vi "Run.vi"(8 "error in (no error)":errorcluster, 11 "Channel in":refnum<class "Channel.lvclass">) -> (0 "error out":errorcluster, 3 "Channel out":refnum<class "Channel.lvclass">)   [LabVIEW 2018, in "Channel.lvclass"]
doc: "Run the channel"
uses:
  Channel.lvclass
  Channel.lvclass/Channel.ctl
  Simulated_CCD_Camera/Simulated Camera.lvclass/Simulated Camera.ctl
  State Machine/State Machine.lvclass
  Simulated_CCD_Camera/Simulated Camera.lvclass
  RxTx/RxTx.lvclass
  Header content/Header content.lvclass
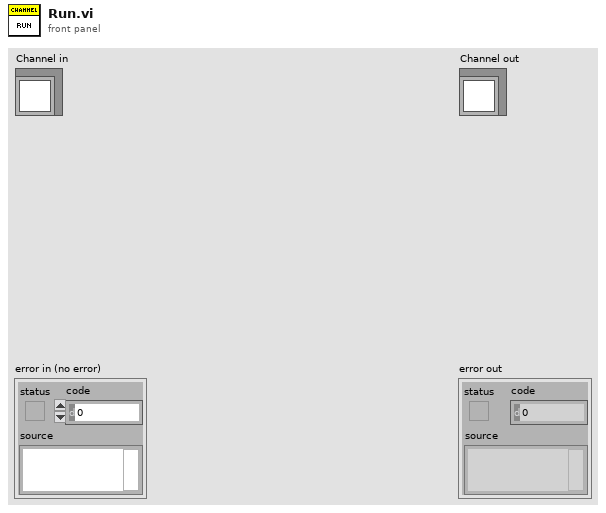
[diagram p1: front panel]
types:
  T1 = cluster{"PREAMP":u16, "READOUT_RATE":u16, "EM_GAIN":u16, "VERTICAL_SHIFT_SPEED":u16, "READ_MODE":u16, "FRAME_TRANSFER":bool, "VERTICAL_CLOCK_VOLTAGE":u16, "ACQUISITION_MODE":u16, "AD_CHANNEL":u16, "EM_MODE":u16, "SHUTTER_TTL":u16, "SHUTTER_OPENING_TIME":u16, "SHUTTER_CLOSING_TIME":u16, "SHUTTER_MODE":u16, "TRIGGER_MODE":u16, "VBIN":u16, "INITIAL_LINE":u16, "INITIAL_COLUMN":u16, "FINAL_LINE":u16, "FINAL_COLUMN":u16, "HBIN":u16}
  T2 = cluster{"CYCLES_DONE":u16, "LAST_IMAGE_NAME":string, "DISK_SPACE":u16, "FRAMES_DONE":u16, "CCD_STATUS":string, "CURRENT_TEMPERATURE":i16, "TEMPERATURE_STATUS":string, "FRAME_EXPOSURE_TIME":sgl, "ERROR":bool, "SERIAL_NUMBER":u16, "ACQUIRING":bool, "IMAGE_INDEX":u32, "SEQS_DONE":u16}
  T3 = cluster{"COOLER_POWER_STATUS":u16, "TEMP":i32, "EXPTIME":dbl, "#FRAMES":u32, "#CYCLES":u32, "#SEQS":u32, "WAVEPLATE_POS":u16}
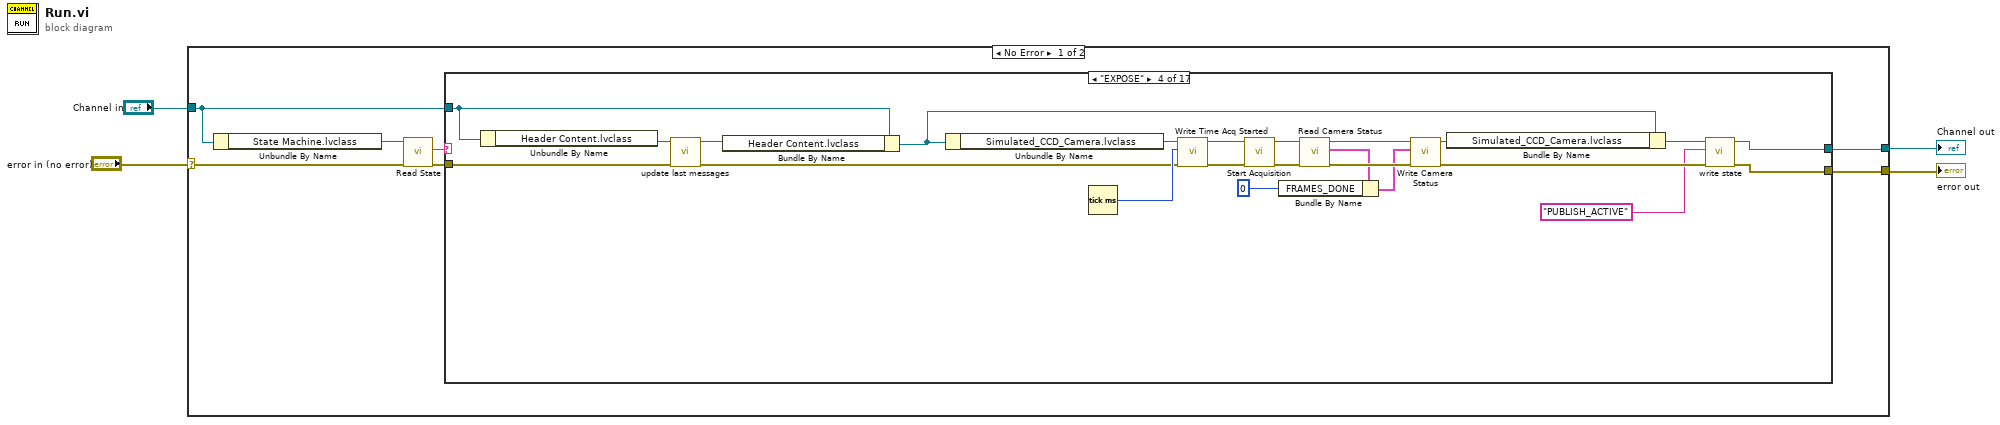
[diagram p0: block diagram]
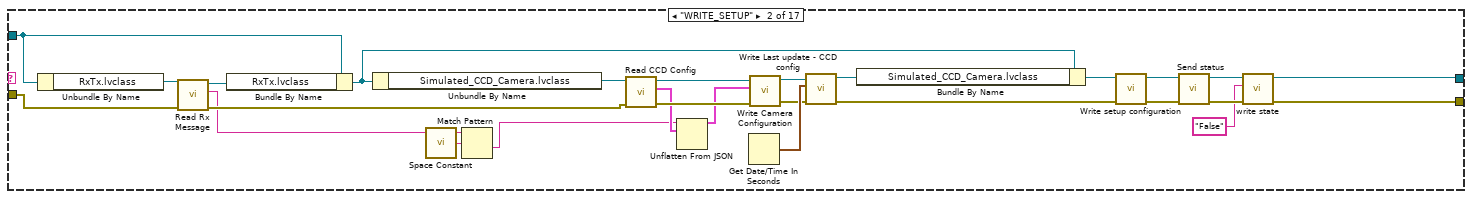
[diagram p3: hidden frame]
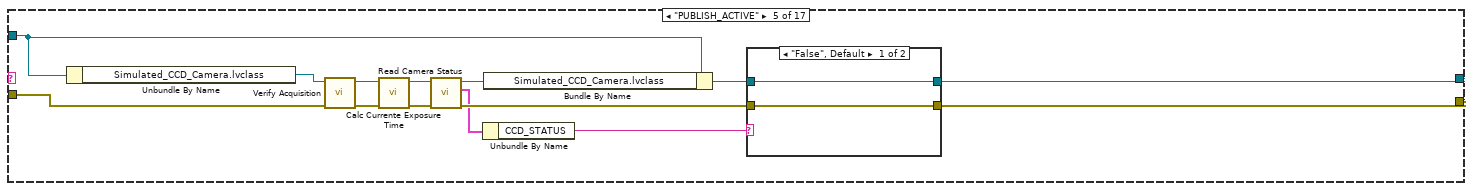
[diagram p5: hidden frame]
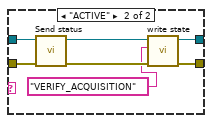
[diagram p6: hidden frame]
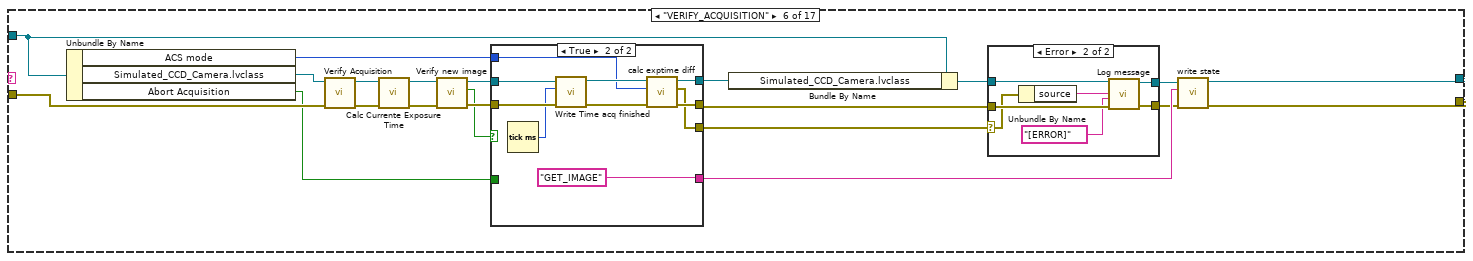
[diagram p7: hidden frame]
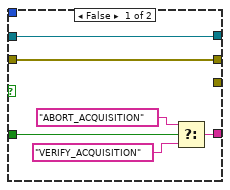
[diagram p9: hidden frame]
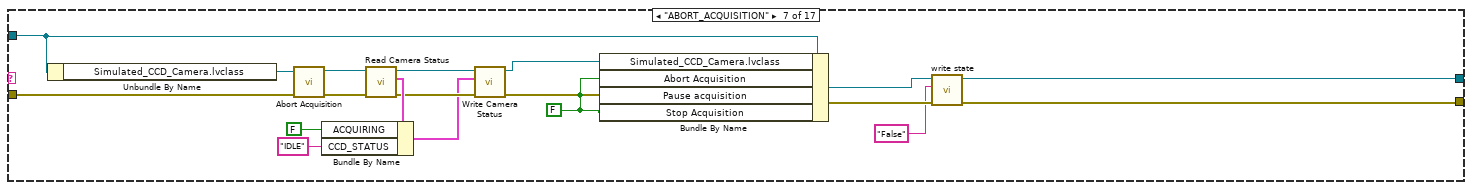
[diagram p10: hidden frame]
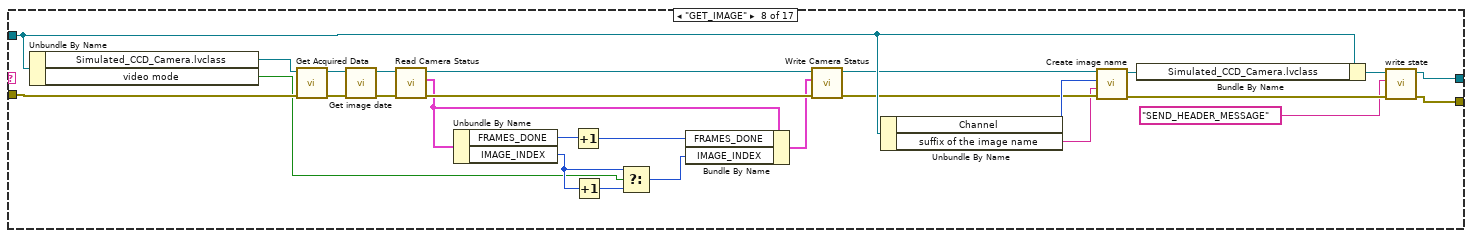
[diagram p11: hidden frame]
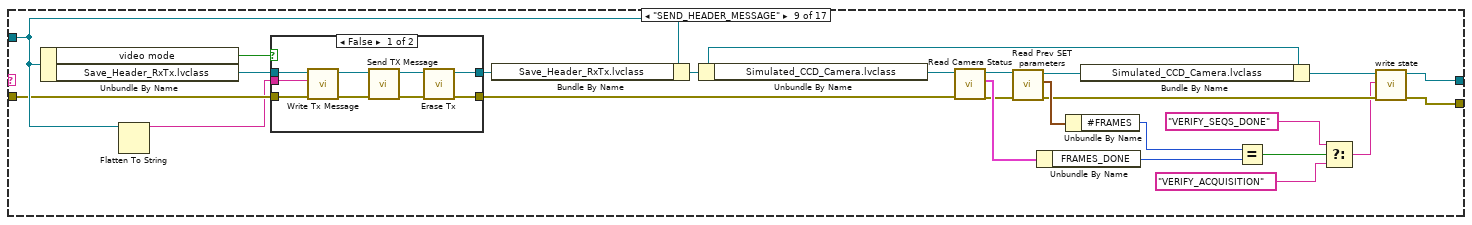
[diagram p12: hidden frame]
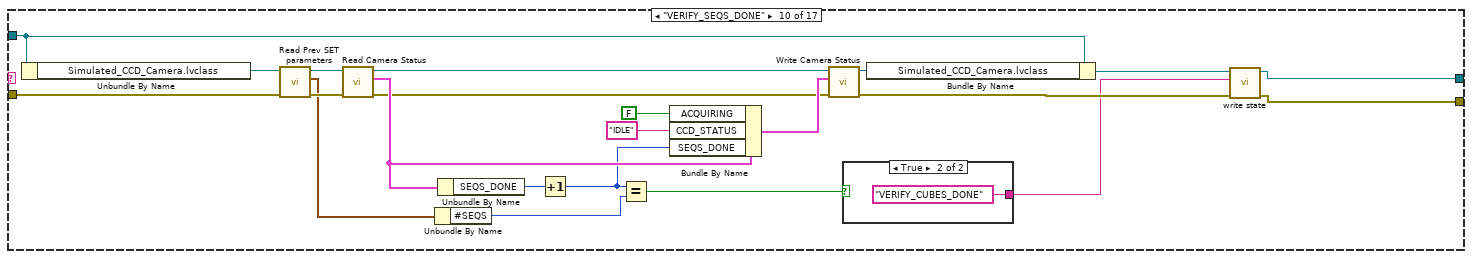
[diagram p14: hidden frame]
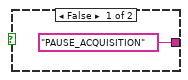
[diagram p15: hidden frame]
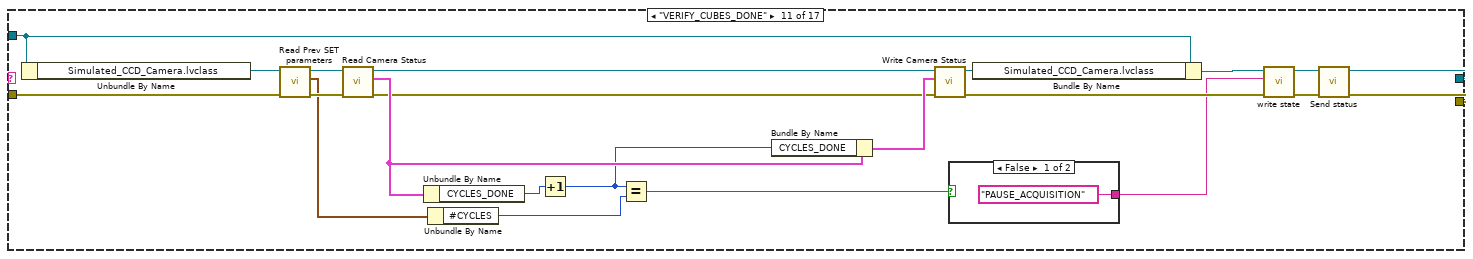
[diagram p16: hidden frame]
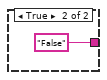
[diagram p17: hidden frame]
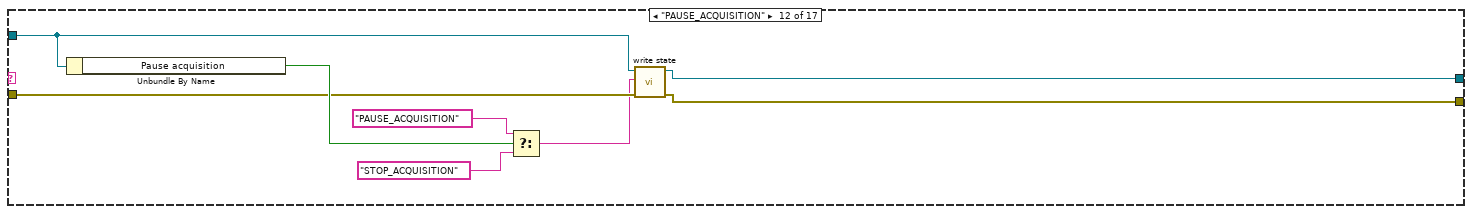
[diagram p18: hidden frame]
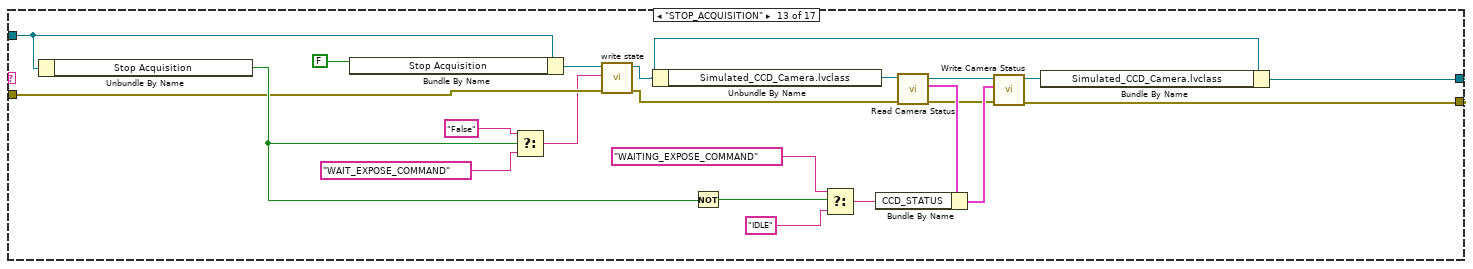
[diagram p19: hidden frame]
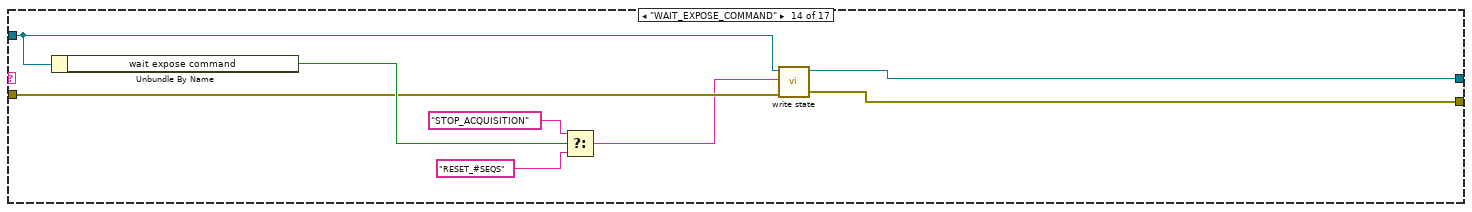
[diagram p20: hidden frame]
diagram:
  n1 = case shown="No Error" "error in (no error)" {
    selector: "error in (no error)" -> [w7 w427]
    tunnel: [w11 w427] -> w3
    tunnel: [w9 w426] -> w1
    tunnel: "Channel in" -> [w10 w426]
    frame No Error {
      n2 = Unbundle By Name(w10) -> ("State Machine.lvclass"=w8:refnum<class "State Machine.lvclass">)
      n3 = call-dynamic "Read State.vi"("error in (no error)"=w7, "State Machine in"=w8) -> ("error out"=w6:errorcluster, "State"=w5:string)  [unwired: 7 in, 1 out]
      n4 = case shown="\"EXPOSE\"" w5 {
        tunnel: w6 -> [w12 w38 w41 w56 w76 w105 w143 w179 w189 w227 w252 w266 w272 w296 w304 w322 w339]
        tunnel: [w12 w23 w41 w47 w72 w101 w136 w153 w180 w215 w244 w265 w279 w295 w301 w322 w329] -> w11
        tunnel: [w13 w24 w42 w48 w73 w102 w137 w154 w181 w216 w245 w264 w280 w294 w302 w323 w330] -> w9
        tunnel: w10 -> [w13 w40 w42 w55 w79 w109 w142 w172 w191 w231 w258 w267 w292 w297 w307 w323 w341]
        frame "False", Default {
        }
        frame "WRITE_SETUP" {
          n5 = Unbundle By Name(w40) -> ("RxTx.lvclass"=w39:refnum<class "RxTx.lvclass">)
          n6 = call "Read Rx Message.vi"("error in (no error)"=w38, "RxTx in"=w39) -> ("error out"=w33:errorcluster, "Rx Message"=w15:string, "RxTx out"=w37:refnum<class "RxTx.lvclass">)  [unwired: 7 in]
          n7 = Bundle By Name(cluster=w40, "RxTx.lvclass"=w37) -> (w28:refnum<class "Channel.lvclass">)
          n8 = Unbundle By Name(w28) -> ("Simulated_CCD_Camera.lvclass"=w36:refnum<class "Simulated Camera.lvclass">)
          n9 = call <vilib>:"Space Constant.vi"() -> ("String"=w16:string)
          n10 = Match Pattern(string=w15, regular expression=w16) -> (after substring=w14:string)  [unwired: 1 in, 3 out]
          n11 = call "Read CCD Config.vi"("error in (no error)"=w33, "CCDCamera in"=w36) -> ("error out"=w34:errorcluster, "CCD Config"=w32:T1, "CCDCamera out"=w35:refnum<class "Simulated Camera.lvclass">)  [unwired: 7 in]
          n12 = Unflatten From JSON(JSON string=w14, type and defaults=w32) -> (value=w31:T1)  [unwired: 5 in, 1 out]
          n13 = Get Date/Time In Seconds() -> (seconds since 1Jan1904=w30:timestamp)
          n14 = call-dynamic "Write Camera Configuration.vi"("error in (no error)"=w34, "CCD Config"=w31, "CCDCamera in"=w35) -> ("error out"=w21:errorcluster, "CCDCamera out"=w22:refnum<class "Simulated Camera.lvclass">)  [unwired: 7 in]
          n15 = call-dynamic "Write Last update - CCD config.vi"("error in (no error)"=w21, "Last update - CCD config"=w30, "Simulated_CCD_Camera in"=w22) -> ("error out"=w19:errorcluster, "Simulated_CCD_Camera out"=w29:refnum<class "Simulated Camera.lvclass">)  [unwired: 7 in]
          n16 = Bundle By Name(cluster=w28, "Simulated_CCD_Camera.lvclass"=w29) -> (w20:refnum<class "Channel.lvclass">)
          n17 = call "Write setup configuration.vi"("error in (no error)"=w19, "Channel in"=w20) -> ("error out"=w18:errorcluster, "Channel out"=w17:refnum<class "Channel.lvclass">)  [unwired: 8 in]
          n18 = call "Send status.vi"("error in (no error)"=w18, "Channel in"=w17) -> ("error out"=w26:errorcluster, "Channel out"=w27:refnum<class "Channel.lvclass">)  [unwired: 8 in]
          n19 = call "write state.vi"("error in (no error)"=w26, "state"="False", "Channel in"=w27) -> ("error out"=w23:errorcluster, "Channel out"=w24:refnum<class "Channel.lvclass">)  [unwired: 7 in]
        }
        frame "---------------------------------" {
        }
        frame "EXPOSE" {
          n20 = Unbundle By Name(w55) -> ("Header Content.lvclass"=w57:refnum<class "Header content.lvclass">)
          n21 = call "update last messages.vi"("error in (no error)"=w56, "Header content in"=w57) -> ("error out"=w53:errorcluster, "Header content out"=w54:refnum<class "Header content.lvclass">)  [unwired: 8 in]
          n22 = Bundle By Name(cluster=w55, "Header Content.lvclass"=w54) -> (w52:refnum<class "Channel.lvclass">)
          n23 = Unbundle By Name(w52) -> ("Simulated_CCD_Camera.lvclass"=w65:refnum<class "Simulated Camera.lvclass">)
          n24 = Tick Count (ms)() -> (millisecond timer value=w64:u32)
          n25 = call "Write Time Acq Started.vi"("error in (no error)"=w53, "Time Acq Started"=w64, "Simulated_CCD_Camera in"=w65) -> ("error out"=w43:errorcluster, "Simulated_CCD_Camera out"=w46:refnum<class "Simulated Camera.lvclass">)  [unwired: 7 in]
          n26 = call-dynamic "Start Acquisition.vi"("error in (no error)"=w43, "CCDCamera in"=w46) -> ("error out"=w44:errorcluster, "CCDCamera out"=w45:refnum<class "Simulated Camera.lvclass">)  [unwired: 8 in]
          n27 = call "Read Camera Status.vi"("error in (no error)"=w44, "CCDCamera in"=w45) -> ("error out"=w62:errorcluster, "Camera Status"=w60:T2, "CCDCamera out"=w61:refnum<class "Simulated Camera.lvclass">)  [unwired: 7 in]
          n28 = Bundle By Name(cluster=w60, "FRAMES_DONE"=u16 0) -> (w59:T2)
          n29 = call "Write Camera Status.vi"("error in (no error)"=w62, "Camera Status"=w59, "CCDCamera in"=w61) -> ("error out"=w50:errorcluster, "CCDCamera out"=w63:refnum<class "Simulated Camera.lvclass">)  [unwired: 7 in]
          n30 = Bundle By Name(cluster=w52, "Simulated_CCD_Camera.lvclass"=w63) -> (w51:refnum<class "Channel.lvclass">)
          n31 = call "write state.vi"("error in (no error)"=w50, "state"="PUBLISH_ACTIVE", "Channel in"=w51) -> ("error out"=w47:errorcluster, "Channel out"=w48:refnum<class "Channel.lvclass">)  [unwired: 7 in]
        }
        frame "PUBLISH_ACTIVE" {
          n32 = Unbundle By Name(w79) -> ("Simulated_CCD_Camera.lvclass"=w77:refnum<class "Simulated Camera.lvclass">)
          n33 = call-dynamic "Verify Acquisition.vi"("error in (no error)"=w76, "CCDCamera in"=w77) -> ("error out"=w78:errorcluster, "CCDCamera out"=w75:refnum<class "Simulated Camera.lvclass">)  [unwired: 8 in]
          n34 = call-dynamic "Calc Currente Exposure Time.vi"("error in (no error)"=w78, "CCDCamera in"=w75) -> ("error out"=w71:errorcluster, "CCDCamera out"=w70:refnum<class "Simulated Camera.lvclass">)  [unwired: 8 in]
          n35 = call "Read Camera Status.vi"("error in (no error)"=w71, "CCDCamera in"=w70) -> ("error out"=w68:errorcluster, "Camera Status"=w67:T2, "CCDCamera out"=w69:refnum<class "Simulated Camera.lvclass">)  [unwired: 7 in]
          n36 = Unbundle By Name(w67) -> ("CCD_STATUS"=w66:string)
          n37 = Bundle By Name(cluster=w79, "Simulated_CCD_Camera.lvclass"=w69) -> (w74:refnum<class "Channel.lvclass">)
          n38 = case shown="\"False\", Default" w66 {
            tunnel: w74 -> [w81 w84]
            tunnel: [w81 w88] -> w73
            tunnel: [w80 w87] -> w72
            tunnel: w68 -> [w80 w83]
            frame "False", Default {
            }
            frame "ACTIVE" {
              n39 = call "Send status.vi"("error in (no error)"=w83, "Channel in"=w84) -> ("error out"=w86:errorcluster, "Channel out"=w85:refnum<class "Channel.lvclass">)  [unwired: 8 in]
              n40 = call "write state.vi"("error in (no error)"=w86, "state"="VERIFY_ACQUISITION", "Channel in"=w85) -> ("error out"=w87:errorcluster, "Channel out"=w88:refnum<class "Channel.lvclass">)  [unwired: 7 in]
            }
          }
        }
        frame "VERIFY_ACQUISITION" {
          n41 = Unbundle By Name(w109) -> ("ACS mode"=w94:u16, "Simulated_CCD_Camera.lvclass"=w106:refnum<class "Simulated Camera.lvclass">, "Abort Acquisition"=w97:bool)
          n42 = call-dynamic "Verify Acquisition.vi"("error in (no error)"=w105, "CCDCamera in"=w106) -> ("error out"=w107:errorcluster, "CCDCamera out"=w104:refnum<class "Simulated Camera.lvclass">)  [unwired: 8 in]
          n43 = call-dynamic "Calc Currente Exposure Time.vi"("error in (no error)"=w107, "CCDCamera in"=w104) -> ("error out"=w108:errorcluster, "CCDCamera out"=w103:refnum<class "Simulated Camera.lvclass">)  [unwired: 8 in]
          n44 = call-dynamic "Verify new image.vi"("error in (no error)"=w108, "CCDCamera in"=w103) -> ("error out"=w99:errorcluster, "New Images ?"=w96:bool, "CCDCamera out"=w100:refnum<class "Simulated Camera.lvclass">)  [unwired: 7 in]
          n45 = case shown="True" w96 {
            tunnel: w100 -> [w124 w134]
            tunnel: w99 -> [w123 w133]
            tunnel: [w124 w128] -> w98
            tunnel: [w123 w129] -> w90
            tunnel: w97 -> [w120 _]
            tunnel: [w119 "GET_IMAGE"] -> w95
            tunnel: w94 -> [_ w126]
            tunnel: [_ w125] -> w89
            frame False {
              n46 = Select(t="ABORT_ACQUISITION", s=w120, f="VERIFY_ACQUISITION") -> (s? t:f=w119:string)
            }
            frame True {
              n47 = Tick Count (ms)() -> (millisecond timer value=w131:u32)
              n48 = call "Write Time acq finished.vi"("error in (no error)"=w133, "Time acq finished"=w131, "Simulated_CCD_Camera in"=w134) -> ("error out"=w130:errorcluster, "Simulated_CCD_Camera out"=w127:refnum<class "Simulated Camera.lvclass">)  [unwired: 7 in]
              n49 = call "calc exptime diff.vi"("error in (no error)"=w130, "ACS mode"=w126, "Simulated_CCD_Camera in"=w127) -> (0:"error out"=w129:errorcluster, 2:"error out"=w125:errorcluster, "Simulated_CCD_Camera out"=w128:refnum<class "Simulated Camera.lvclass">)  [unwired: 6 in]
            }
          }
          n50 = Bundle By Name(cluster=w109, "Simulated_CCD_Camera.lvclass"=w98) -> (w93:refnum<class "Channel.lvclass">)
          n51 = case shown="Error" w89 {
            selector: w89 -> [_ w113]
            tunnel: w93 -> [w111 w118]
            tunnel: [w111 w117] -> w92
            tunnel: [w110 w116] -> w91
            tunnel: w90 -> [w110 w115]
            frame No Error {
            }
            frame Error {
              n52 = Unbundle By Name(w113) -> ("source"=w112:string)
              n53 = call "Log message.vi"("error in (no error)"=w115, "message type"="[ERROR]", "String"=w112, "Channel in"=w118) -> ("error out"=w116:errorcluster, "Channel out"=w117:refnum<class "Channel.lvclass">)  [unwired: 6 in]
            }
          }
          n54 = call "write state.vi"("error in (no error)"=w91, "state"=w95, "Channel in"=w92) -> ("error out"=w101:errorcluster, "Channel out"=w102:refnum<class "Channel.lvclass">)  [unwired: 7 in]
        }
        frame "ABORT_ACQUISITION" {
          w135 = FALSE ("Acquiring")
          n55 = Unbundle By Name(w142) -> ("Simulated_CCD_Camera.lvclass"=w144:refnum<class "Simulated Camera.lvclass">)
          n56 = call-dynamic "Abort Acquisition.vi"("error in (no error)"=w143, "CCDCamera in"=w144) -> ("error out"=w149:errorcluster, "CCDCamera out"=w150:refnum<class "Simulated Camera.lvclass">)  [unwired: 8 in]
          n57 = call "Read Camera Status.vi"("error in (no error)"=w149, "CCDCamera in"=w150) -> ("error out"=w147:errorcluster, "Camera Status"=w152:T2, "CCDCamera out"=w148:refnum<class "Simulated Camera.lvclass">)  [unwired: 7 in]
          n58 = Bundle By Name(cluster=w152, "ACQUIRING"=FALSE ("Acquiring"), "CCD_STATUS"="IDLE" ("STATUS")) -> (w146:T2)
          n59 = call "Write Camera Status.vi"("error in (no error)"=w147, "Camera Status"=w146, "CCDCamera in"=w148) -> ("error out"=w139:errorcluster, "CCDCamera out"=w141:refnum<class "Simulated Camera.lvclass">)  [unwired: 7 in]
          n60 = Bundle By Name(cluster=w142, "Simulated_CCD_Camera.lvclass"=w141, "Abort Acquisition"=w135, "Pause acquisition"=w135, "Stop Acquisition"=w135) -> (w140:refnum<class "Channel.lvclass">)
          n61 = call "write state.vi"("error in (no error)"=w139, "state"="False", "Channel in"=w140) -> ("error out"=w136:errorcluster, "Channel out"=w137:refnum<class "Channel.lvclass">)  [unwired: 7 in]
        }
        frame "GET_IMAGE" {
          n62 = Unbundle By Name(w172) -> ("Simulated_CCD_Camera.lvclass"=w161:refnum<class "Simulated Camera.lvclass">, "video mode"=w158:bool)
          n63 = call-dynamic "Get Acquired Data.vi"("error in (no error)"=w179, "CCDCamera in"=w161) -> ("error out"=w164:errorcluster, "CCDCamera out"=w167:refnum<class "Simulated Camera.lvclass">)  [unwired: 8 in]
          n64 = call-dynamic "Get image date.vi"("error in (no error)"=w164, "Simulated_CCD_Camera in"=w167) -> ("error out"=w165:errorcluster, "Simulated_CCD_Camera out"=w166:refnum<class "Simulated Camera.lvclass">)  [unwired: 8 in]
          n65 = call "Read Camera Status.vi"("error in (no error)"=w165, "CCDCamera in"=w166) -> ("error out"=w178:errorcluster, "Camera Status"=w174:T2, "CCDCamera out"=w177:refnum<class "Simulated Camera.lvclass">)  [unwired: 7 in]
          n66 = Unbundle By Name(w174) -> ("FRAMES_DONE"=w176:u16, "IMAGE_INDEX"=w159:u32)
          n67 = Increment(x=w176) -> (x+1=w162:u16)
          n68 = Increment(x=w159) -> (x+1=w160:u32)
          n69 = Select(t=w159, s=w158, f=w160) -> (s? t:f=w163:u32)
          n70 = Bundle By Name(cluster=w174, "FRAMES_DONE"=w162, "IMAGE_INDEX"=w163) -> (w175:T2)
          n71 = call "Write Camera Status.vi"("error in (no error)"=w178, "Camera Status"=w175, "CCDCamera in"=w177) -> ("error out"=w169:errorcluster, "CCDCamera out"=w170:refnum<class "Simulated Camera.lvclass">)  [unwired: 7 in]
          n72 = Unbundle By Name(w172) -> ("Channel"=w171:u8, "suffix of the image name"=w168:string)
          n73 = call "Create image name.vi"("error in (no error)"=w169, "Suffix"=w168, "Channel"=w171, "Simulated_CCD_Camera in"=w170) -> ("error out"=w156:errorcluster, "Simulated_CCD_Camera out"=w173:refnum<class "Simulated Camera.lvclass">)  [unwired: 6 in]
          n74 = Bundle By Name(cluster=w172, "Simulated_CCD_Camera.lvclass"=w173) -> (w157:refnum<class "Channel.lvclass">)
          n75 = call "write state.vi"("error in (no error)"=w156, "state"="SEND_HEADER_MESSAGE", "Channel in"=w157) -> ("error out"=w153:errorcluster, "Channel out"=w154:refnum<class "Channel.lvclass">)  [unwired: 7 in]
        }
        frame "SEND_HEADER_MESSAGE" {
          n76 = Unbundle By Name(w191) -> ("video mode"=w185:bool, "Save_Header_RxTx.lvclass"=w190:refnum<class "RxTx.lvclass">)
          n77 = Flatten To String(anything=w191) -> (data string=w186:string)  [unwired: 3 in, 2 out]
          n78 = case shown="False" w185 {
            tunnel: w190 -> [w212 w214]
            tunnel: w189 -> [w209 w213]
            tunnel: [w207 w214] -> w188
            tunnel: [w205 w213] -> w187
            tunnel: w186 -> [w204 _]
            frame False {
              n79 = call "Write Tx Message.vi"("error in (no error)"=w209, "Tx Message"=w204, "RxTx in"=w212) -> ("error out"=w210:errorcluster, "RxTx out"=w211:refnum<class "RxTx.lvclass">)  [unwired: 7 in]
              n80 = call "Send TX Message.vi"("error in (no error)"=w210, "RxTx in"=w211) -> ("error out"=w206:errorcluster, "RxTx out"=w208:refnum<class "RxTx.lvclass">)  [unwired: 8 in]
              n81 = call "Erase Tx.vi"("error in (no error)"=w206, "RxTx in"=w208) -> ("error out"=w205:errorcluster, "RxTx out"=w207:refnum<class "RxTx.lvclass">)  [unwired: 8 in]
            }
            frame True {
            }
          }
          n82 = Bundle By Name(cluster=w191, "Save_Header_RxTx.lvclass"=w188) -> (w201:refnum<class "Channel.lvclass">)
          n83 = Unbundle By Name(w201) -> ("Simulated_CCD_Camera.lvclass"=w198:refnum<class "Simulated Camera.lvclass">)
          n84 = call "Read Camera Status.vi"("error in (no error)"=w187, "CCDCamera in"=w198) -> ("error out"=w194:errorcluster, "Camera Status"=w197:T2, "CCDCamera out"=w196:refnum<class "Simulated Camera.lvclass">)  [unwired: 7 in]
          n85 = call-dynamic "Read Prev SET parameters.vi"("error in (no error)"=w194, "Simulated_CCD_Camera in"=w196) -> ("error out"=w183:errorcluster, "Prev SET parameters"=w193:T3, "Simulated_CCD_Camera out"=w195:refnum<class "Simulated Camera.lvclass">)  [unwired: 7 in]
          n86 = Unbundle By Name(w197) -> ("FRAMES_DONE"=w203:u16)
          n87 = Unbundle By Name(w193) -> ("#FRAMES"=w192:u32)
          n88 = Bundle By Name(cluster=w201, "Simulated_CCD_Camera.lvclass"=w195) -> (w184:refnum<class "Channel.lvclass">)
          n89 = Equal?(x=w192, y=w203) -> (x = y?=w202:bool)
          n90 = Select(t="VERIFY_SEQS_DONE", s=w202, f="VERIFY_ACQUISITION") -> (s? t:f=w182:string)
          n91 = call "write state.vi"("error in (no error)"=w183, "state"=w182, "Channel in"=w184) -> ("error out"=w180:errorcluster, "Channel out"=w181:refnum<class "Channel.lvclass">)  [unwired: 7 in]
        }
        frame "VERIFY_SEQS_DONE" {
          n92 = Unbundle By Name(w231) -> ("Simulated_CCD_Camera.lvclass"=w230:refnum<class "Simulated Camera.lvclass">)
          n93 = call-dynamic "Read Prev SET parameters.vi"("error in (no error)"=w227, "Simulated_CCD_Camera in"=w230) -> ("error out"=w228:errorcluster, "Prev SET parameters"=w226:T3, "Simulated_CCD_Camera out"=w229:refnum<class "Simulated Camera.lvclass">)  [unwired: 7 in]
          n94 = call "Read Camera Status.vi"("error in (no error)"=w228, "CCDCamera in"=w229) -> ("error out"=w222:errorcluster, "Camera Status"=w236:T2, "CCDCamera out"=w223:refnum<class "Simulated Camera.lvclass">)  [unwired: 7 in]
          n95 = Unbundle By Name(w226) -> ("#SEQS"=w225:u32)
          n96 = Unbundle By Name(w236) -> ("SEQS_DONE"=w235:u16)
          n97 = Increment(x=w235) -> (x+1=w233:u16)
          n98 = Equal?(x=w233, y=w225) -> (x = y?=w232:bool)
          n99 = Bundle By Name(cluster=w236, "ACQUIRING"=FALSE, "CCD_STATUS"="IDLE", "SEQS_DONE"=w233) -> (w234:T2)
          n100 = call "Write Camera Status.vi"("error in (no error)"=w222, "Camera Status"=w234, "CCDCamera in"=w223) -> ("error out"=w218:errorcluster, "CCDCamera out"=w224:refnum<class "Simulated Camera.lvclass">)  [unwired: 7 in]
          n101 = case shown="True" w232 {
            tunnel: ["PAUSE_ACQUISITION" "VERIFY_CUBES_DONE"] -> w217
            frame False {
            }
            frame True {
            }
          }
          n102 = Bundle By Name(cluster=w231, "Simulated_CCD_Camera.lvclass"=w224) -> (w219:refnum<class "Channel.lvclass">)
          n103 = call "write state.vi"("error in (no error)"=w218, "state"=w217, "Channel in"=w219) -> ("error out"=w215:errorcluster, "Channel out"=w216:refnum<class "Channel.lvclass">)  [unwired: 7 in]
        }
        frame "VERIFY_CUBES_DONE" {
          n104 = Unbundle By Name(w258) -> ("Simulated_CCD_Camera.lvclass"=w255:refnum<class "Simulated Camera.lvclass">)
          n105 = call-dynamic "Read Prev SET parameters.vi"("error in (no error)"=w252, "Simulated_CCD_Camera in"=w255) -> ("error out"=w253:errorcluster, "Prev SET parameters"=w251:T3, "Simulated_CCD_Camera out"=w254:refnum<class "Simulated Camera.lvclass">)  [unwired: 7 in]
          n106 = call "Read Camera Status.vi"("error in (no error)"=w253, "CCDCamera in"=w254) -> ("error out"=w256:errorcluster, "Camera Status"=w260:T2, "CCDCamera out"=w257:refnum<class "Simulated Camera.lvclass">)  [unwired: 7 in]
          n107 = Unbundle By Name(w260) -> ("CYCLES_DONE"=w246:u16)
          n108 = Unbundle By Name(w251) -> ("#CYCLES"=w250:u32)
          n109 = Increment(x=w246) -> (x+1=w248:u16)
          n110 = Equal?(x=w248, y=w250) -> (x = y?=w247:bool)
          n111 = Bundle By Name(cluster=w260, "CYCLES_DONE"=w248) -> (w259:T2)
          n112 = call "Write Camera Status.vi"("error in (no error)"=w256, "Camera Status"=w259, "CCDCamera in"=w257) -> ("error out"=w240:errorcluster, "CCDCamera out"=w249:refnum<class "Simulated Camera.lvclass">)  [unwired: 7 in]
          n113 = case shown="False" w247 {
            tunnel: ["PAUSE_ACQUISITION" "False"] -> w239
            frame False {
            }
            frame True {
            }
          }
          n114 = Bundle By Name(cluster=w258, "Simulated_CCD_Camera.lvclass"=w249) -> (w243:refnum<class "Channel.lvclass">)
          n115 = call "write state.vi"("error in (no error)"=w240, "state"=w239, "Channel in"=w243) -> ("error out"=w241:errorcluster, "Channel out"=w242:refnum<class "Channel.lvclass">)  [unwired: 7 in]
          n116 = call "Send status.vi"("error in (no error)"=w241, "Channel in"=w242) -> ("error out"=w244:errorcluster, "Channel out"=w245:refnum<class "Channel.lvclass">)  [unwired: 8 in]
        }
        frame "PAUSE_ACQUISITION" {
          n117 = Unbundle By Name(w267) -> ("Pause acquisition"=w270:bool)
          n118 = Select(t="PAUSE_ACQUISITION", s=w270, f="STOP_ACQUISITION") -> (s? t:f=w263:string)
          n119 = call "write state.vi"("error in (no error)"=w266, "state"=w263, "Channel in"=w267) -> ("error out"=w265:errorcluster, "Channel out"=w264:refnum<class "Channel.lvclass">)  [unwired: 7 in]
        }
        frame "STOP_ACQUISITION" {
          n120 = Unbundle By Name(w292) -> ("Stop Acquisition"=w276:bool)
          n121 = Bundle By Name(cluster=w292, "Stop Acquisition"=FALSE) -> (w275:refnum<class "Channel.lvclass">)
          n122 = Select(t="False", s=w276, f="WAIT_EXPOSE_COMMAND") -> (s? t:f=w271:string)
          n123 = call "write state.vi"("error in (no error)"=w272, "state"=w271, "Channel in"=w275) -> ("error out"=w273:errorcluster, "Channel out"=w274:refnum<class "Channel.lvclass">)  [unwired: 7 in]
          n124 = Unbundle By Name(w274) -> ("Simulated_CCD_Camera.lvclass"=w288:refnum<class "Simulated Camera.lvclass">)
          n125 = Not(x=w276) -> (.not. x?=w277:bool)
          n126 = Select(t="WAITING_EXPOSE_COMMAND" ("CCD_STATUS"), s=w277, f="IDLE" ("CCD_STATUS")) -> (s? t:f=w282:string)
          n127 = call "Read Camera Status.vi"("error in (no error)"=w273, "CCDCamera in"=w288) -> ("error out"=w285:errorcluster, "Camera Status"=w287:T2, "CCDCamera out"=w284:refnum<class "Simulated Camera.lvclass">)  [unwired: 7 in]
          n128 = Bundle By Name(cluster=w287, "CCD_STATUS"=w282) -> (w286:T2)
          n129 = call "Write Camera Status.vi"("error in (no error)"=w285, "Camera Status"=w286, "CCDCamera in"=w284) -> ("error out"=w279:errorcluster, "CCDCamera out"=w283:refnum<class "Simulated Camera.lvclass">)  [unwired: 7 in]
          n130 = Bundle By Name(cluster=w274, "Simulated_CCD_Camera.lvclass"=w283) -> (w280:refnum<class "Channel.lvclass">)
        }
        frame "WAIT_EXPOSE_COMMAND" {
          n131 = Unbundle By Name(w297) -> ("wait expose command"=w298:bool)
          n132 = Select(t="STOP_ACQUISITION", s=w298, f="RESET_#SEQS") -> (s? t:f=w293:string)
          n133 = call "write state.vi"("error in (no error)"=w296, "state"=w293, "Channel in"=w297) -> ("error out"=w295:errorcluster, "Channel out"=w294:refnum<class "Channel.lvclass">)  [unwired: 7 in]
        }
        frame "RESET_#SEQS" {
          n134 = call "write state.vi"("error in (no error)"=w304, "state"="EXPOSE", "Channel in"=w307) -> ("error out"=w305:errorcluster, "Channel out"=w306:refnum<class "Channel.lvclass">)  [unwired: 7 in]
          n135 = Unbundle By Name(w306) -> ("Simulated_CCD_Camera.lvclass"=w318:refnum<class "Simulated Camera.lvclass">)
          n136 = call "Read Camera Status.vi"("error in (no error)"=w305, "CCDCamera in"=w318) -> ("error out"=w311:errorcluster, "Camera Status"=w319:T2, "CCDCamera out"=w310:refnum<class "Simulated Camera.lvclass">)  [unwired: 7 in]
          n137 = call-dynamic "Read Prev SET parameters.vi"("error in (no error)"=w311, "Simulated_CCD_Camera in"=w310) -> ("error out"=w308:errorcluster, "Prev SET parameters"=w317:T3, "Simulated_CCD_Camera out"=w309:refnum<class "Simulated Camera.lvclass">)  [unwired: 7 in]
          n138 = Unbundle By Name(w319) -> ("SEQS_DONE"=w313:u16)
          n139 = Unbundle By Name(w317) -> ("#SEQS"=w316:u32)
          n140 = Equal?(x=w313, y=w316) -> (x = y?=w315:bool)
          n141 = Select(t=0, s=w315, f=w313) -> (s? t:f=w312:i32)
          n142 = Bundle By Name(cluster=w319, "SEQS_DONE"=w312) -> (w321:T2)
          n143 = call "Write Camera Status.vi"("error in (no error)"=w308, "Camera Status"=w321, "CCDCamera in"=w309) -> ("error out"=w301:errorcluster, "CCDCamera out"=w320:refnum<class "Simulated Camera.lvclass">)  [unwired: 7 in]
          n144 = Bundle By Name(cluster=w306, "Simulated_CCD_Camera.lvclass"=w320) -> (w302:refnum<class "Channel.lvclass">)
        }
        frame "------------------------------" {
        }
        frame "SET" {
          n145 = Unbundle By Name(w341) -> ("RxTx.lvclass"=w338:refnum<class "RxTx.lvclass">)
          n146 = call "Read Rx Message.vi"("error in (no error)"=w339, "RxTx in"=w338) -> ("error out"=w340:errorcluster, "Rx Message"=w336:string)  [unwired: 7 in, 1 out]
          n147 = call <vilib>:"Space Constant.vi"() -> ("String"=w335:string)
          n148 = Match Pattern(string=w336, regular expression=w335) -> (after substring=w337:string)  [unwired: 1 in, 3 out]
          n149 = Match Pattern(string=w337, regular expression=w335) -> (before substring=w334:string, after substring=w333:string)  [unwired: 1 in, 2 out]
          n150 = case shown="\"SUFFIX\"" w334 {
            tunnel: [w343 w355 w368 w381 w393 w406 w419 w424] -> w325
            tunnel: w341 -> [w343 w356 w369 w382 w394 w407 w420 w425]
            tunnel: [w342 w348 w361 w374 w383 w399 w412 w423] -> w324
            tunnel: w340 -> [w342 w350 w363 w376 w391 w401 w414 w423]
            tunnel: w333 -> [_ w352 w365 w378 w385 w403 w416 w421]
            frame "False", Default {
            }
            frame "EXPTIME" {
              n151 = Unbundle By Name(w356) -> ("Simulated_CCD_Camera.lvclass"=w351:refnum<class "Simulated Camera.lvclass">)
              n152 = Fract/Exp String To Number(string=w352, default (0 dbl)=0.0) -> (number=w353:dbl)  [unwired: 2 in, 1 out]
              n153 = call-dynamic "Read SET parameters.vi"("error in (no error)"=w350, "Simulated_CCD_Camera in"=w351) -> ("error out"=w344:errorcluster, "New SET parameters"=w347:T3, "Simulated_CCD_Camera out"=w345:refnum<class "Simulated Camera.lvclass">)  [unwired: 7 in]
              n154 = Bundle By Name(cluster=w347, "EXPTIME"=w353) -> (w346:T3)
              n155 = call-dynamic "Write SET parameters.vi"("error in (no error)"=w344, "New SET parameters"=w346, "Simulated_CCD_Camera in"=w345) -> ("error out"=w348:errorcluster, "Simulated_CCD_Camera out"=w349:refnum<class "Simulated Camera.lvclass">)  [unwired: 7 in]
              n156 = Bundle By Name(cluster=w356, "Simulated_CCD_Camera.lvclass"=w349) -> (w355:refnum<class "Channel.lvclass">)
            }
            frame "#FRAMES" {
              n157 = Unbundle By Name(w369) -> ("Simulated_CCD_Camera.lvclass"=w364:refnum<class "Simulated Camera.lvclass">)
              n158 = Fract/Exp String To Number(string=w365, default (0 dbl)=u32 0) -> (number=w366:u32)  [unwired: 2 in, 1 out]
              n159 = call-dynamic "Read SET parameters.vi"("error in (no error)"=w363, "Simulated_CCD_Camera in"=w364) -> ("error out"=w357:errorcluster, "New SET parameters"=w360:T3, "Simulated_CCD_Camera out"=w358:refnum<class "Simulated Camera.lvclass">)  [unwired: 7 in]
              n160 = Bundle By Name(cluster=w360, "#FRAMES"=w366) -> (w359:T3)
              n161 = call-dynamic "Write SET parameters.vi"("error in (no error)"=w357, "New SET parameters"=w359, "Simulated_CCD_Camera in"=w358) -> ("error out"=w361:errorcluster, "Simulated_CCD_Camera out"=w362:refnum<class "Simulated Camera.lvclass">)  [unwired: 7 in]
              n162 = Bundle By Name(cluster=w369, "Simulated_CCD_Camera.lvclass"=w362) -> (w368:refnum<class "Channel.lvclass">)
            }
            frame "#CYCLES" {
              n163 = Unbundle By Name(w382) -> ("Simulated_CCD_Camera.lvclass"=w377:refnum<class "Simulated Camera.lvclass">)
              n164 = Fract/Exp String To Number(string=w378, default (0 dbl)=u32 0) -> (number=w379:u32)  [unwired: 2 in, 1 out]
              n165 = call-dynamic "Read SET parameters.vi"("error in (no error)"=w376, "Simulated_CCD_Camera in"=w377) -> ("error out"=w370:errorcluster, "New SET parameters"=w373:T3, "Simulated_CCD_Camera out"=w371:refnum<class "Simulated Camera.lvclass">)  [unwired: 7 in]
              n166 = Bundle By Name(cluster=w373, "#CYCLES"=w379) -> (w372:T3)
              n167 = call-dynamic "Write SET parameters.vi"("error in (no error)"=w370, "New SET parameters"=w372, "Simulated_CCD_Camera in"=w371) -> ("error out"=w374:errorcluster, "Simulated_CCD_Camera out"=w375:refnum<class "Simulated Camera.lvclass">)  [unwired: 7 in]
              n168 = Bundle By Name(cluster=w382, "Simulated_CCD_Camera.lvclass"=w375) -> (w381:refnum<class "Channel.lvclass">)
            }
            frame "WAVEPLATE_POS" {
              n169 = Unbundle By Name(w394) -> ("Simulated_CCD_Camera.lvclass"=w392:refnum<class "Simulated Camera.lvclass">)
              n170 = Decimal String To Number(string=w385) -> (number=w386:i32)  [unwired: 2 in, 1 out]
              n171 = call-dynamic "Read SET parameters.vi"("error in (no error)"=w391, "Simulated_CCD_Camera in"=w392) -> ("error out"=w387:errorcluster, "New SET parameters"=w390:T3, "Simulated_CCD_Camera out"=w388:refnum<class "Simulated Camera.lvclass">)  [unwired: 7 in]
              n172 = Bundle By Name(cluster=w390, "WAVEPLATE_POS"=w386) -> (w389:T3)
              n173 = call-dynamic "Write SET parameters.vi"("error in (no error)"=w387, "New SET parameters"=w389, "Simulated_CCD_Camera in"=w388) -> ("error out"=w383:errorcluster, "Simulated_CCD_Camera out"=w384:refnum<class "Simulated Camera.lvclass">)  [unwired: 7 in]
              n174 = Bundle By Name(cluster=w394, "Simulated_CCD_Camera.lvclass"=w384) -> (w393:refnum<class "Channel.lvclass">)
            }
            frame "TEMP" {
              n175 = Unbundle By Name(w407) -> ("Simulated_CCD_Camera.lvclass"=w402:refnum<class "Simulated Camera.lvclass">)
              n176 = Fract/Exp String To Number(string=w403, default (0 dbl)=0) -> (number=w404:i32)  [unwired: 2 in, 1 out]
              n177 = call-dynamic "Read SET parameters.vi"("error in (no error)"=w401, "Simulated_CCD_Camera in"=w402) -> ("error out"=w395:errorcluster, "New SET parameters"=w398:T3, "Simulated_CCD_Camera out"=w396:refnum<class "Simulated Camera.lvclass">)  [unwired: 7 in]
              n178 = Bundle By Name(cluster=w398, "TEMP"=w404) -> (w397:T3)
              n179 = call-dynamic "Write SET parameters.vi"("error in (no error)"=w395, "New SET parameters"=w397, "Simulated_CCD_Camera in"=w396) -> ("error out"=w399:errorcluster, "Simulated_CCD_Camera out"=w400:refnum<class "Simulated Camera.lvclass">)  [unwired: 7 in]
              n180 = Bundle By Name(cluster=w407, "Simulated_CCD_Camera.lvclass"=w400) -> (w406:refnum<class "Channel.lvclass">)
            }
            frame "COOLER_POWER_STATUS" {
              n181 = Unbundle By Name(w420) -> ("Simulated_CCD_Camera.lvclass"=w415:refnum<class "Simulated Camera.lvclass">)
              n182 = Fract/Exp String To Number(string=w416, default (0 dbl)=u16 0) -> (number=w417:u16)  [unwired: 2 in, 1 out]
              n183 = call-dynamic "Read SET parameters.vi"("error in (no error)"=w414, "Simulated_CCD_Camera in"=w415) -> ("error out"=w408:errorcluster, "New SET parameters"=w411:T3, "Simulated_CCD_Camera out"=w409:refnum<class "Simulated Camera.lvclass">)  [unwired: 7 in]
              n184 = Bundle By Name(cluster=w411, "COOLER_POWER_STATUS"=w417) -> (w410:T3)
              n185 = call-dynamic "Write SET parameters.vi"("error in (no error)"=w408, "New SET parameters"=w410, "Simulated_CCD_Camera in"=w409) -> ("error out"=w412:errorcluster, "Simulated_CCD_Camera out"=w413:refnum<class "Simulated Camera.lvclass">)  [unwired: 7 in]
              n186 = Bundle By Name(cluster=w420, "Simulated_CCD_Camera.lvclass"=w413) -> (w419:refnum<class "Channel.lvclass">)
            }
            frame "SUFFIX" {
              n187 = To Lower Case(string=w421) -> (all lower case string=w422:string)
              n188 = Bundle By Name(cluster=w425, "suffix of the image name"=w422) -> (w424:refnum<class "Channel.lvclass">)
            }
          }
          n189 = call "Write acquisition configuration.vi"("error in (no error)"=w324, "Channel in"=w325) -> ("error out"=w327:errorcluster, "Channel out"=w326:refnum<class "Channel.lvclass">)  [unwired: 8 in]
          n190 = call "Send status.vi"("error in (no error)"=w327, "Channel in"=w326) -> ("error out"=w331:errorcluster, "Channel out"=w332:refnum<class "Channel.lvclass">)  [unwired: 8 in]
          n191 = call "write state.vi"("error in (no error)"=w331, "state"="False", "Channel in"=w332) -> ("error out"=w329:errorcluster, "Channel out"=w330:refnum<class "Channel.lvclass">)  [unwired: 7 in]
        }
      }
    }
    frame Error {
    }
  }
  "error out" <- w3
  "Channel out" <- w1
